vi "globalTearDown.vi"(8 "error in (no error)":errorcluster, 11 "testcase-CSMArgument in":refnum<class "testcase-CSMArgument.lvclass">) -> (0 "error out":errorcluster, 3 "testcase-CSMArgument out":refnum<class "testcase-CSMArgument.lvclass">)   [LabVIEW 2017, in "testcase-CSMArgument.lvclass"]
uses:
  testcase-CSMArgument.lvclass
  testcase-CSMArgument.lvclass/testcase-CSMArgument.ctl
  <vilib>/addons/_JKI Toolkits/VI Tester/TestCase.llb/TestCase.lvclass
  src/user.lib/_NEVSTOP/Communicable State Machine(CSM)/Communicable State Machine.lvlib
  src/user.lib/_NEVSTOP/Communicable State Machine(CSM)/_Support/Typedef/_CSM_List Module Scope.ctl
panel:
  out "Module Names":string[](array[string])
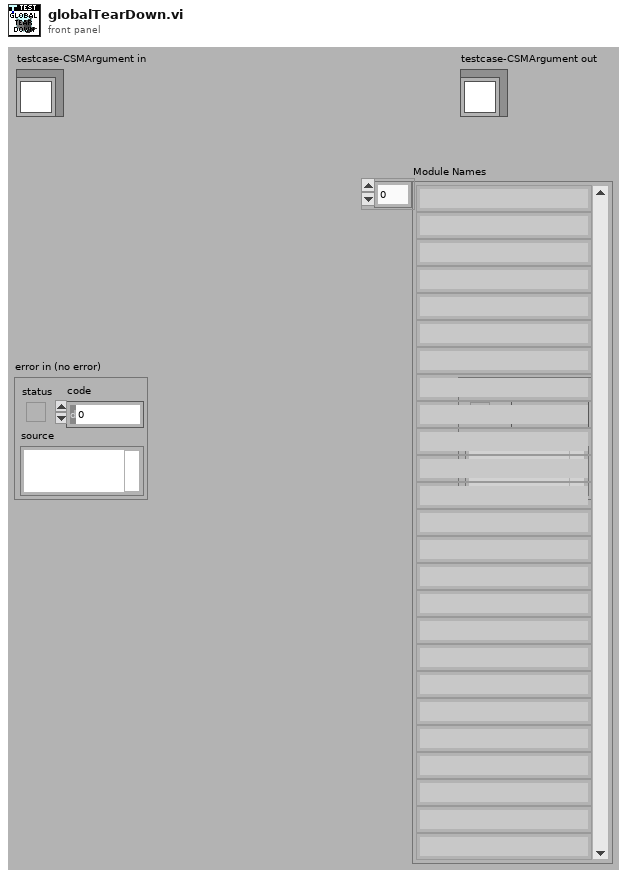
[diagram p1: front panel]
types:
  T1 = typedef "Communicable State Machine.lvlib/_CSM_List Module Scope.ctl" = enum16{"Normal", "System Only", "All"}
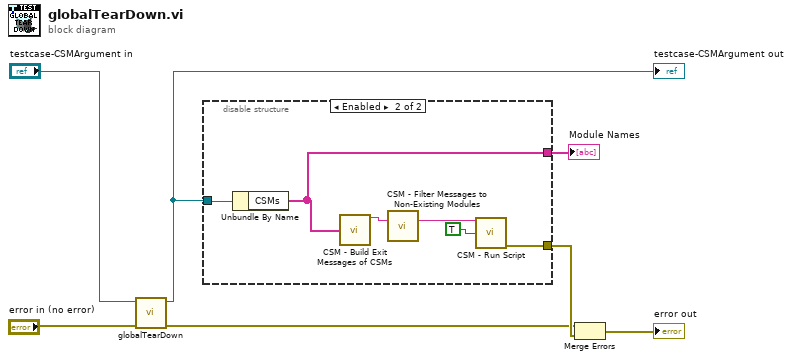
[diagram p0: block diagram]
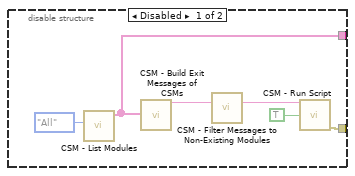
[diagram p2: hidden frame]
diagram:
  n1 = call-parent "globalTearDown.vi"("error in (no error)"="error in (no error)", "TestCase in"="testcase-CSMArgument in") -> ("error out"=w4:errorcluster, "TestCase out"=w1:refnum<class "testcase-CSMArgument.lvclass">)  [unwired: 8 in]
  "testcase-CSMArgument out" <- w1
  n2 = disable-structure shown="Enabled" {
    disable-tunnel: [w9 w14] -> w6
    disable-tunnel: w1 -> [_ w19]
    disable-tunnel: [w8 w15] -> w3
    frame Disabled {
      n3 = call "CSM - List Modules.vi"("Scope (Normal)"=_CSM_List_Module_Scope."All") -> ("Module Names"=w8:string[])  [unwired: 9 in, 1 out]
      n4 = call "CSM - Build Exit Messages of CSMs.vi"("CSMs"=w8) -> ("States"=w13:string)  [unwired: 14 in]
      n5 = call "CSM - Filter Messages to Non-Existing Modules.vi"("States In"=w13) -> ("States Out"=w11:string)  [unwired: 14 in]
      n6 = call "CSM - Run Script.vi"("CSM Scripts"=w11, "Continue If Error? (F)"=TRUE) -> ("error out"=w9:errorcluster)  [unwired: 11 in, 2 out]
    }
    frame Enabled {
      n7 = Unbundle By Name(w19) -> ("CSMs"=w15:string[])
      n8 = call "CSM - Build Exit Messages of CSMs.vi"("CSMs"=w15) -> ("States"=w18:string)  [unwired: 14 in]
      n9 = call "CSM - Filter Messages to Non-Existing Modules.vi"("States In"=w18) -> ("States Out"=w16:string)  [unwired: 14 in]
      n10 = call "CSM - Run Script.vi"("CSM Scripts"=w16, "Continue If Error? (F)"=TRUE) -> ("error out"=w14:errorcluster)  [unwired: 11 in, 2 out]
    }
  }
  "Module Names" <- w3
  n11 = Merge Errors(w4, w6) -> (→"error out":errorcluster)
